vi "login.vi"() -> (0 "Corret":bool)   [LabVIEW 2014]
panel:
  in  "Username":string
  in  "Password":string
  in  "Stop Button":bool
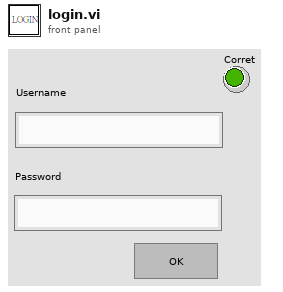
[diagram p1: front panel]
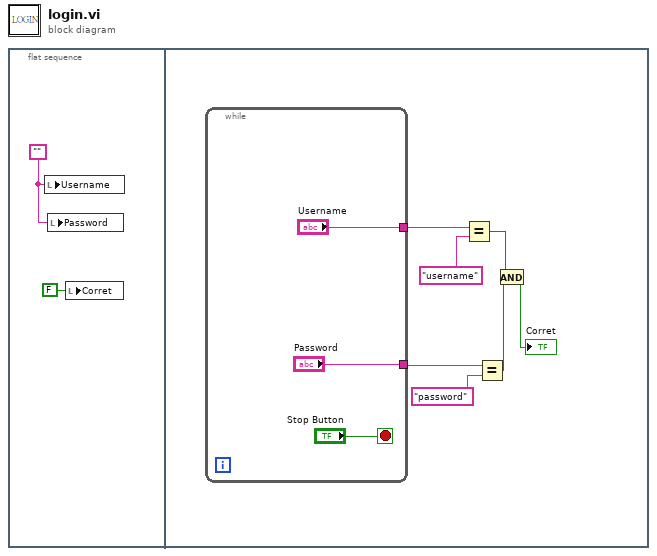
[diagram p0: block diagram]
diagram:
  n1 = flat-sequence {
    frame #0 {
      w2 = ""
      n2 = local write "Username"(w2) -> ()
      n3 = local write "Password"(w2) -> ()
      n4 = local write "Corret"(FALSE ("Corret")) -> ()
    }
    frame #1 {
      n5 = while {
        tunnel: ["Username"] -> w5
        tunnel: ["Password"] -> w4
        stop <- "Stop Button" stop-if-true
      }
      n6 = Equal?(x=w5, y="username") -> (x = y?=w7:bool)
      n7 = Equal?(x=w4, y="password") -> (x = y?=w8:bool)
      n8 = And(x=w7, y=w8) -> (x .and. y?=→"Corret":bool)
    }
  }
